vi "Query Multi Eval Meas List Segment DMRS Type A.vi"(0 "VISA resource name":refnum<visa-resource-name>, 1 "BWP (0)":i32, 5 "Instance (1)":T2=1, 7 "Segment (1)":i32=1, 9 "CC (1)":T1=1, 11 "error in (no error)":errorcluster) -> (4 "VISA resource name out":refnum<visa-resource-name>, 6 "Config Type":i32, 8 "Additional Position":i32, 10 "Max Length":i32, 15 "error out":errorcluster)   [LabVIEW 2020, in "Rohde&Schwarz CMWXP NR FR1 Measurement.lvlib"]
doc: "Queries the DM-RS for mapping type A. The settings apply to the <BWP> on carrier <cc> in segment <no>.\n\nAttribute:\n-\n\nRemote-control command:\nCONFigure:NRSub:MEAS<i>:LIST:SEGMent<no>[:CC<cc>]:BWPart:PUSCh:DMTA?"
uses:
  <instrlib>/Rohde&Schwarz CMWXP NR FR1 Measurement/Rohde&Schwarz CMWXP NR FR1 Measurement.lvlib
  <instrlib>/Rohde&Schwarz CMWXP NR FR1 Measurement/Private/_Instance.ctl
  <instrlib>/Rohde&Schwarz CMWXP NR FR1 Measurement/Private/_Carrier Component.ctl
  <instrlib>/Rohde&Schwarz CMWXP NR FR1 Measurement/Private/rsidr_core.llb/rsidr_core.lvlib
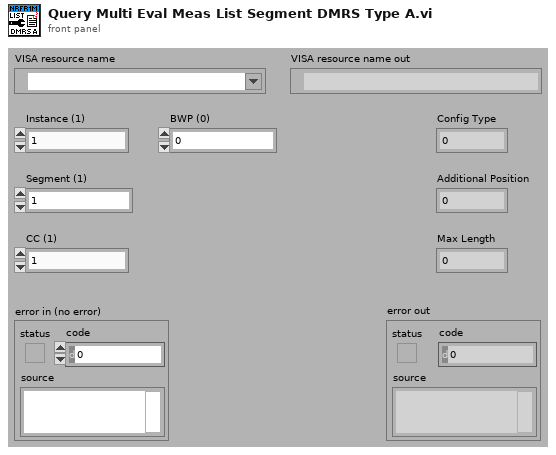
[diagram p1: front panel]
types:
  T1 = typedef "Rohde&Schwarz CMWXP NR FR1 Measurement.lvlib/_Carrier Component.ctl" = i32
  T2 = typedef "Rohde&Schwarz CMWXP NR FR1 Measurement.lvlib/_Instance.ctl" = i32
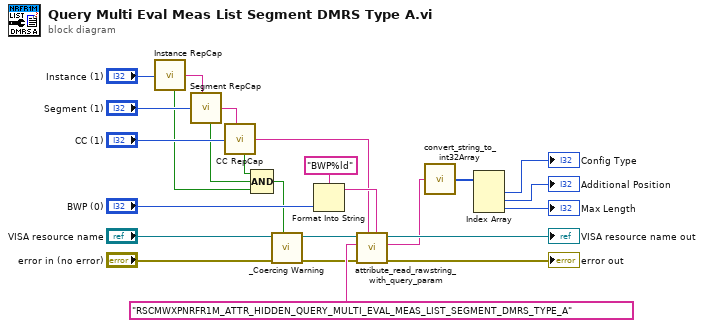
[diagram p0: block diagram]
diagram:
  n1 = call <instrlib>:"Instance RepCap.vi"("Instance In"="Instance (1)") -> ("In Range?"=w3:bool, "RepCap Identifier Out"=w21:string)  [unwired: 1 in]
  n2 = call <instrlib>:"Segment RepCap.vi"("Segment In"="Segment (1)", "RepCap String In (\"\")"=w21) -> ("In Range?"=w2:bool, "RepCap Identifier Out"=w22:string)
  n3 = call <instrlib>:"CC RepCap.vi"("CC In"="CC (1)", "RepCap String In (\"\")"=w22) -> ("In Range?"=w1:bool, "RepCap Identifier Out"=w15:string)
  n4 = Compound Arithmetic op=AND(w1, w2, w3) -> (w4:bool)
  n5 = call <instrlib>:"_Coercing Warning.vi"("In Range?"=w4, "error in (no error)"="error in (no error)", "VISA resource name"="VISA resource name") -> ("error out"=w6:errorcluster, "VISA resource name out"=w5:refnum<visa-resource-name>)  [unwired: 7 in]
  n6 = Format Into String(format string="BWP%ld", "BWP (0)") -> (resulting string=w16:string)  [unwired: 2 in, 1 out]
  n7 = call <instrlib>:"attribute_read_rawstring_with_query_param.vi"("Query Parameter (None)"=w16, "Repeated Capability"=w15, "error in"=w6, "Attribute ID"="RSCMWXPNRFR1M_ATTR_HIDDEN_QUERY_MULTI_EVAL_MEAS_LIST_SEGMENT_DMRS_TYPE_A", "VISA resource name"=w5) -> ("error out"=→"error out":errorcluster, "Raw String out"=w13:string, "VISA resource name out"=→"VISA resource name out":refnum<visa-resource-name>)  [unwired: 4 in]
  n8 = call <instrlib>:"convert_string_to_int32Array.vi"("string in"=w13) -> ("int32 array out"=w12:i32[])  [unwired: 3 in, 1 out]
  n9 = Index Array(array=w12) -> (element #1=→"Config Type":i32, element #2=→"Additional Position":i32, element #3=→"Max Length":i32)  [unwired: 3 in]
